vi "TPKT - Write Packet.vi"(8 "error in":errorcluster, 10 "TPDU":T1 format="0x%02x", 11 "S7":refnum<class "S7NetCom.lvclass">) -> (0 "error out":errorcluster, 3 "S7 out":refnum<class "S7NetCom.lvclass">)   [LabVIEW 2014, in "S7NetCom.lvclass"]
doc: "Writes the TPKT packet to the network.\n\n_____\nCopyright (c) 2019 Hampel Software Engineering (HSE), released under BSD license. More info can be found on https://dokuwiki.hampel-soft.com/code/hse/s7netcom. Original code published by Marc Christenson, Sisu Devices."
uses:
  S7NetCom.lvclass
  Controls/S7NetCom_HexByteArray.ctl
  Controls/S7NetCom_HexByte.ctl
  S7NetCom.lvclass/S7NetCom.ctl
  TPKT - Header Bytes 1 and 2--constant.vi
panel:
  # "More info on https://dokuwiki.hampel-soft.com/code/hse/s7netcom\n\nCopyright (c) 2019, HAMPEL SOFTWARE ENGINEERING (HSE)\nOriginal code developed by Marc Christenson, Sisu Devices\nAll rights reserved.\n\nRedistribution and use in source and binary forms, with or without\nmodification, are permitted provided that the following conditions are met:\n\n1. Redistributions of source code must retain the above copyright\n   notice, this list of conditions and the following disclaimer.\n\n2. Redistributions in binary form must reproduce the above copyright\n   notice, this list of conditions and the following disclaimer in the\n   documentation and/or other materials provided with the distribution.\n\n3. All advertising materials mentioning features or use of this software\n   must display the following acknowledgement:\n   This product includes software developed by HAMPEL SOFTWARE ENGINEERING.\n\n4. Neither the name of HAMPEL SOFTWARE ENGINEERING nor the\n   names of its contributors may be used to endorse or promote products\n   derived from this software without specific prior written permission.\n\nTHIS SOFTWARE IS PROVIDED BY HAMPEL SOFTWARE ENGINEERING ''AS IS'' AND ANY\nEXPRESS OR IMPLIED WARRANTIES, INCLUDING, BUT NOT LIMITED TO, THE IMPLIED\nWARRANTIES OF MERCHANTABILITY AND FITNESS FOR A PARTICULAR PURPOSE ARE\nDISCLAIMED. IN NO EVENT SHALL HAMPEL SOFTWARE ENGINEERING BE LIABLE FOR ANY\nDIRECT, INDIRECT, INCIDENTAL, SPECIAL, EXEMPLARY, OR CONSEQUENTIAL DAMAGES\n(INCLUDING, BUT NOT LIMITED TO, PROCUREMENT OF SUBSTITUTE GOODS OR SERVICES;\nLOSS OF USE, DATA, OR PROFITS; OR BUSINESS INTERRUPTION) HOWEVER CAUSED AND\nON ANY THEORY OF LIABILITY, WHETHER IN CONTRACT, STRICT LIABILITY, OR TORT\n(INCLUDING NEGLIGENCE OR OTHERWISE) ARISING IN ANY WAY OUT OF THE USE OF THIS\nSOFTWARE, EVEN IF ADVISED OF THE POSSIBILITY OF SUCH DAMAGE."
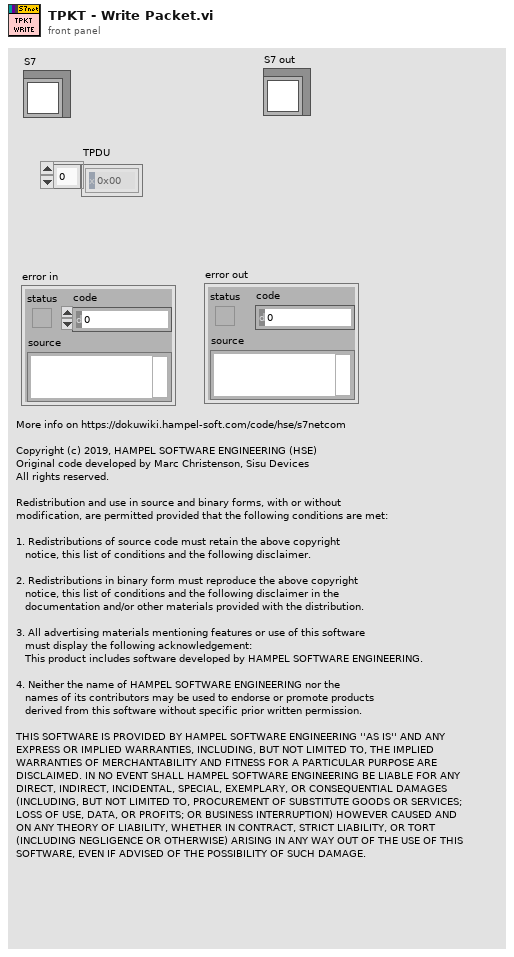
[diagram p1: front panel]
types:
  T1 = typedef "S7NetCom.lvclass/S7NetCom_HexByteArray.ctl" = T2[]
  T2 = typedef "S7NetCom.lvclass/S7NetCom_HexByte.ctl" = u8
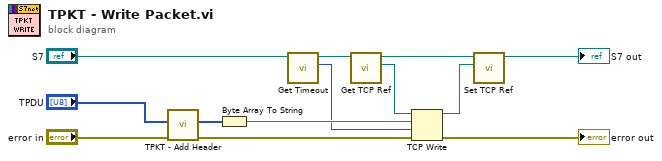
[diagram p0: block diagram]
diagram:
  n1 = call "TPKT - Add Header.vi"("error in (no error)"="error in", "TPDU"="TPDU") -> ("error out"=w10:errorcluster, "TPKT"=w11:T1)  [unwired: 8 in]
  n2 = Byte Array To String(unsigned byte array=w11) -> (string=w13:string)
  n3 = call "Get Timeout.vi"("S7NetCom in"="S7") -> ("Timeout [ms]"=w8:i32, "S7NetCom out"=w4:refnum<class "S7NetCom.lvclass">)  [unwired: 9 in]
  n4 = call "Get TCP Ref.vi"("S7NetCom in"=w4) -> ("TCP Ref"=w2:refnum<k5>, "S7NetCom out"=w3:refnum<class "S7NetCom.lvclass">)  [unwired: 9 in]
  n5 = TCP Write(connection ID=w2, data in=w13, error in (no error)=w10, 9:w8) -> (connection ID out=w5:refnum<k5>, error out=→"error out":errorcluster)  [unwired: 1 out]
  n6 = call "Set TCP Ref.vi"("TCP Ref"=w5, "S7NetCom in"=w3) -> ("S7NetCom out"=→"S7 out":refnum<class "S7NetCom.lvclass">)  [unwired: 9 in]
